vi "test Add-Find-Remove Bus Controller.vi"(8 "error in":errorcluster, 11 "TestCase in":refnum<class "Scripting.lvclass">) -> (0 "error out":errorcluster, 3 "TestCase out":refnum<class "Scripting.lvclass">)   [LabVIEW 2020, in "Scripting.lvclass"]
uses:
  Scripting.lvclass
  <vilib>/addons/_JKI Toolkits/VI Tester/TestCase.llb/TestCase.lvclass
  Scripting/Ballard MIL-STD-1553 Scripting.lvlib
  <vilib>/NI VeriStand/Custom Device API/Custom Device Item Ref.ctl
  <vilib>/NI VeriStand/Custom Device API/Custom Device API.lvlib
  C:/Program Files (x86)/National Instruments/LabVIEW 2020/vi.lib/addons/_JKI Toolkits/VI Tester/TestCase.llb/TestCase.lvclass
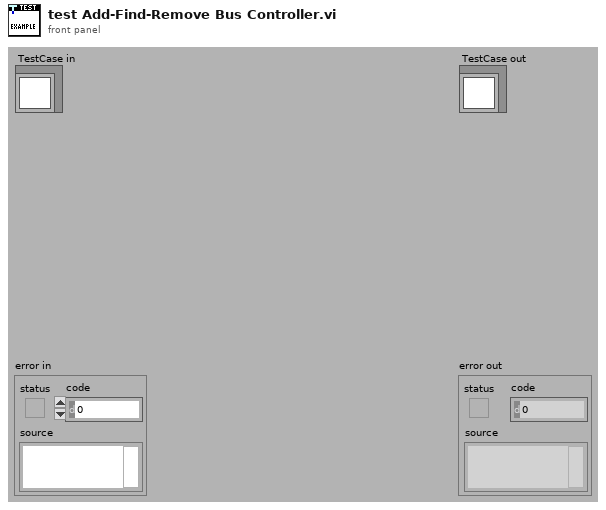
[diagram p1: front panel]
types:
  T1 = typedef "Custom Device API.lvlib/Custom Device Item Ref.ctl" = u64
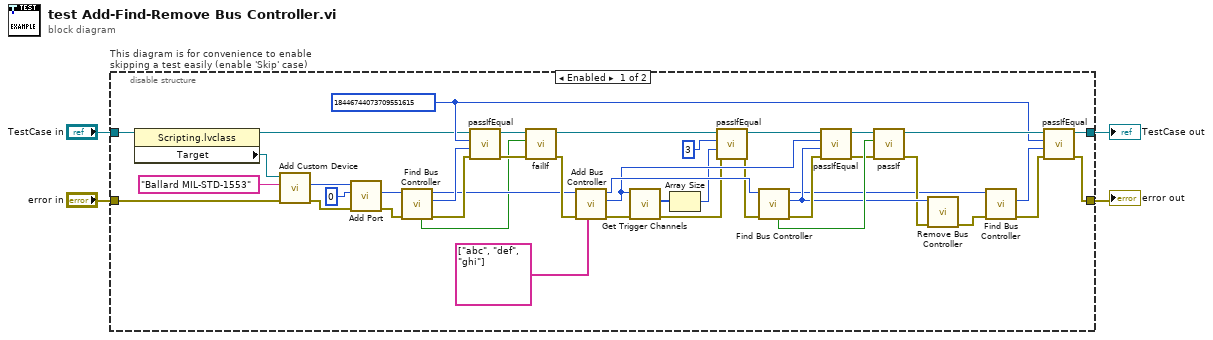
[diagram p0: block diagram]
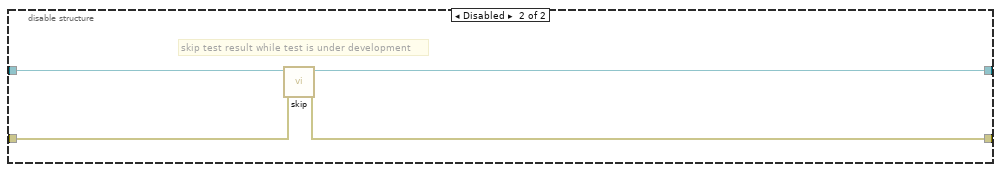
[diagram p2: hidden frame]
diagram:
  n1 = disable-structure "This diagram is for convenience to enable skipping a test easily (enable 'Skip' case)" shown="Enabled" {
    disable-tunnel: "TestCase in" -> [w44 w50]
    disable-tunnel: [w39 w48] -> w1
    disable-tunnel: [w40 w49] -> w3
    disable-tunnel: "error in" -> [w46 w47]
    frame Enabled {
      w22 = T1 18446744073709551615 ("bus controller")
      n2 = property class="Scripting.lvclass"(reference=w44) -> (reference out=w18:refnum<class "Scripting.lvclass">, "Target"=w43:refnum<k24>)  [unwired: 1 in, 1 out]
      n3 = call "Add Custom Device.vi"("error in"=w46, "name"="Ballard MIL-STD-1553", "target in"=w43) -> ("error out"=w37:errorcluster, "Ballard MIL-STD 1553 custom device"=w36:T1)  [unwired: 6 in, 1 out]
      n4 = call "Add Port.vi"("error in"=w37, "port number"=u16 0, "Ballard MIL-STD 1553 custom device in"=w36) -> ("error out"=w34:errorcluster, "port"=w35:T1)  [unwired: 6 in, 1 out]
      n5 = call "Find Bus Controller.vi"("error in"=w34, "port in"=w35) -> ("error out"=w32:errorcluster, "bus controller"=w30:T1, "port out"=w17:T1, "found?"=w16:bool)  [unwired: 6 in]
      n6 = call-dynamic "passIfEqual.vi"("error in (no error)"=w32, "y"=w30, "x"=w22, "TestCase in"=w18) -> ("error out"=w31:errorcluster, "TestCase out"=w19:refnum<class "Scripting.lvclass">)  [unwired: 6 in]
      n7 = call-dynamic "failIf.vi"("error in (no error)"=w31, "fail"=w16, "TestCase in"=w19) -> ("error out"=w33:errorcluster, "TestCase out"=w11:refnum<class "Scripting.lvclass">)  [unwired: 7 in]
      n8 = call "Add Bus Controller.vi"("acyclic frame names"=string[] ["abc", "def", "ghi"], "error in"=w33, "port in"=w17) -> ("error out"=w14:errorcluster, "bus controller"=w12:T1, "port out"=w13:T1)  [unwired: 6 in]
      n9 = call "Get Trigger Channels.vi"("error in"=w14, "acyclic frames section in"=w12) -> ("error out"=w9:errorcluster, "acyclic frame triggers"=w7:T1[])  [unwired: 6 in, 2 out]
      n10 = Array Size(array=w7) -> (size(s)=w6:i32)
      n11 = call-dynamic "passIfEqual.vi"("error in (no error)"=w9, "y"=w6, "x"=3 ("size(s)"), "TestCase in"=w11) -> ("error out"=w8:errorcluster, "TestCase out"=w10:refnum<class "Scripting.lvclass">)  [unwired: 6 in]
      n12 = call "Find Bus Controller.vi"("error in"=w8, "port in"=w13) -> ("error out"=w29:errorcluster, "bus controller"=w26:T1, "port out"=w23:T1, "found?"=w28:bool)  [unwired: 6 in]
      n13 = call-dynamic "passIfEqual.vi"("error in (no error)"=w29, "y"=w26, "x"=w12, "TestCase in"=w10) -> ("error out"=w27:errorcluster, "TestCase out"=w41:refnum<class "Scripting.lvclass">)  [unwired: 6 in]
      n14 = call-dynamic "passIf.vi"("error in (no error)"=w27, "pass"=w28, "TestCase in"=w41) -> ("error out"=w25:errorcluster, "TestCase out"=w38:refnum<class "Scripting.lvclass">)  [unwired: 7 in]
      n15 = call "Remove Bus Controller.vi"("error in"=w25, "bus controller"=w26) -> ("error out"=w24:errorcluster)  [unwired: 9 in]
      n16 = call "Find Bus Controller.vi"("error in"=w24, "port in"=w23) -> ("error out"=w20:errorcluster, "bus controller"=w21:T1)  [unwired: 6 in, 2 out]
      n17 = call-dynamic "passIfEqual.vi"("error in (no error)"=w20, "y"=w21, "x"=w22, "TestCase in"=w38) -> ("error out"=w40:errorcluster, "TestCase out"=w39:refnum<class "Scripting.lvclass">)  [unwired: 6 in]
    }
    frame Disabled {
      # "skip test result while test is under development"
      n18 = call <vilib>:"skip.vi"("error in (no error)"=w47, "TestCase in"=w50) -> ("error out"=w49:errorcluster, "TestCase out"=w48:refnum<class "Scripting.lvclass">)  [unwired: 8 in]
    }
  }
  "error out" <- w3
  "TestCase out" <- w1
